vi "_script_change_copyright_year.vi"(8 "error in (no error)":errorcluster, 11 "dup path":path) -> (0 "error out":errorcluster)   [LabVIEW 2017]
uses:
  _csmHelper/CSM-Helper.lvclass/CSM-Helper.ctl
  _csmHelper/Properties/Read While Loop Ref.vi
  _csmHelper/Utility/Is CSM Module - VIRef.vi
  _csmHelper/API/Create From Basic Refs.vi
  _csmHelper/API/Open Front Panel.vi
  _csmHelper/API/Save Instrument.vi
  _csmHelper/API/Destroy.vi
  _csmHelper/Utility/CSM-Helper Utility.lvlib
  _csmHelper/CSM-Helper.lvclass
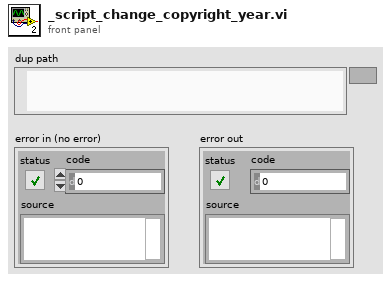
[diagram p1: front panel]
types:
  T1 = typedef "CSM-Helper Utility.lvlib/CSM Basic Refs.ctl" = cluster{"VI":refnum<vi>, "While Loop":refnum<vi>, "Case Structure":refnum<vi>, "Parse State Queue":refnum<vi>, "Event Structure":refnum<vi>, "Type":T2}
  T2 = typedef "CSM-Helper Utility.lvlib/CSM Module Type.ctl" = enum16{"Not a CSM", "JKISM", "CSM"}
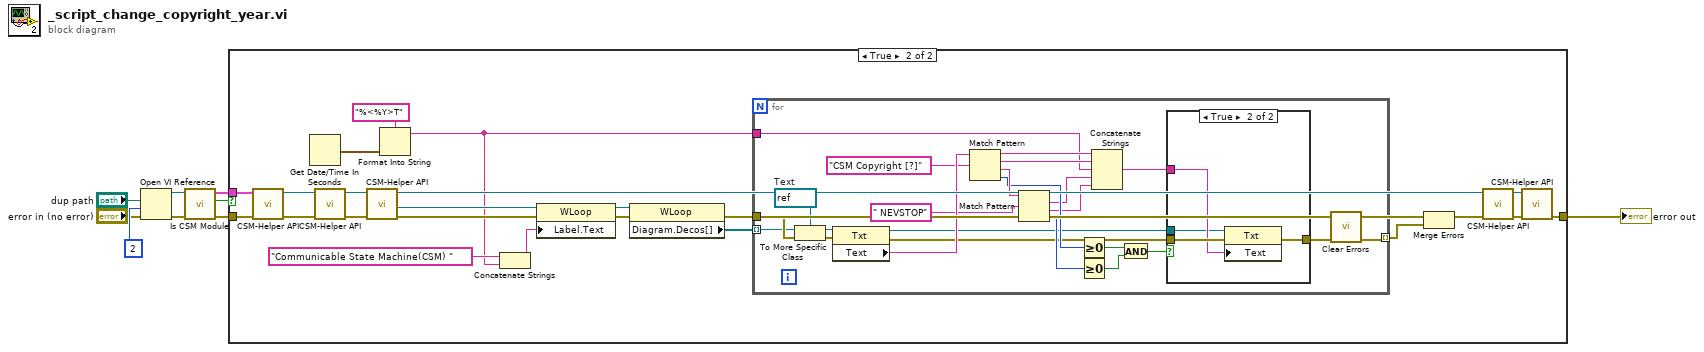
[diagram p0: block diagram]
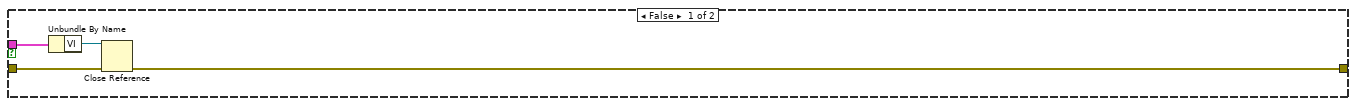
[diagram p2: hidden frame]
diagram:
  n1 = Open VI Reference(vi path="dup path", options=2, error in (no error)="error in (no error)") -> (vi reference=w6:refnum<vi>, error out=w7:errorcluster)  [unwired: 3 in]
  n2 = call-poly "Is CSM Module.vi"("error in (no error)"=w7, "VIRef"=w6) -> ("error out"=w5:errorcluster, "Is CSM Module?"=w8:bool, "CSM Basic Refs"=w4:T1)  [unwired: 7 in]
  n3 = case shown="True" w8 {
    tunnel: [w12 w36] -> w3
    tunnel: w4 -> [w11 w35]
    tunnel: w5 -> [w13 w34]
    frame False {
      n4 = Unbundle By Name(w11) -> ("VI"=w10:refnum<vi>)
      n5 = Close Reference(reference=w10, error in (no error)=w13) -> (error out=w12:errorcluster)
    }
    frame True {
      n6 = call-poly "CSM-Helper API.vi"("error in (no error)"=w34, "CSM Basic Refs"=w35) -> ("error out"=w28:errorcluster, "CSM-Helper.lvclass"=w29:refnum<class "CSM-Helper.lvclass">)  [unwired: 8 in]
      n7 = Get Date/Time In Seconds() -> (seconds since 1Jan1904=w31:timestamp)
      n8 = call-poly "CSM-Helper API.vi"("error in (no error)"=w28, "CSM-Helper in"=w29) -> ("error out"=w27:errorcluster, "CSM-Helper out"=w26:refnum<class "CSM-Helper.lvclass">)  [unwired: 8 in]
      n9 = call-poly "CSM-Helper API.vi"("error in (no error)"=w27, "CSM-Helper in"=w26) -> ("error out"=w33:errorcluster, "While Loop"=w32:refnum<vi>, "CSM-Helper out"=w22:refnum<class "CSM-Helper.lvclass">)  [unwired: 7 in]
      n10 = Format Into String(format string="%<%Y>T", w31) -> (resulting string=w14:string)  [unwired: 2 in, 1 out]
      n11 = Concatenate Strings("Communicable State Machine(CSM) " ("string"), w14) -> (w16:string)
      n12 = property class="WLoop"(reference=w32, error in=w33, "Label.Text"=w16) -> (reference out=w21:refnum<vi>, error out=w23:errorcluster)
      n13 = property class="WLoop"(reference=w21, error in=w23) -> (error out=w20:errorcluster, "Diagram.Decos[]"=w19:refnum<vi>[])  [unwired: 1 out]
      n14 = for {
        tunnel: w20 -> [w60]
        tunnel: w19 -> [w59] mode=indexing
        tunnel: [w55] -> w17 mode=indexing
        tunnel: w14 -> [w42]
        w58 = refnum<vi> refnum  # Text
        n15 = To More Specific Class(target class=w58, reference=w59, error in=w60) -> (specific class reference=w57:refnum<vi>, error out=w56:errorcluster)
        n16 = property class="Txt"(reference=w57, error in=w56) -> (reference out=w37:refnum<vi>, error out=w46:errorcluster, "Text"=w54:string)
        n17 = Match Pattern(string=w54, regular expression="CSM Copyright [?]") -> (before substring=w44:string, match substring=w43:string, after substring=w52:string, offset past match=w50:i32)  [unwired: 1 in]
        n18 = Match Pattern(string=w52, regular expression=" NEVSTOP") -> (match substring=w41:string, after substring=w40:string, offset past match=w49:i32)  [unwired: 1 in, 1 out]
        n19 = Greater Or Equal To 0?(x=w50) -> (x >= 0?=w48:bool)
        n20 = Greater Or Equal To 0?(x=w49) -> (x >= 0?=w47:bool)
        n21 = Concatenate Strings(w44, w43, w42, w41, w40) -> (w39:string)
        n22 = And(x=w48, y=w47) -> (x .and. y?=w38:bool)
        n23 = case shown="True" w38 {
          tunnel: w46 -> [w61 w65]
          tunnel: [w61 w64] -> w45
          tunnel: w39 -> [_ w63]
          tunnel: w37 -> [_ w62]
          frame False {
          }
          frame True {
            n24 = property class="Txt"(reference=w62, error in=w65, "Text"=w63) -> (error out=w64:errorcluster)  [unwired: 1 out]
          }
        }
        n25 = call <vilib>:"Clear Errors.vi"("error in (no error)"=w45) -> ("error out"=w55:errorcluster)  [unwired: 5 in, 1 out]
      }
      n26 = Merge Errors(w20, w17) -> (w18:errorcluster)
      n27 = call-poly "CSM-Helper API.vi"("error in (no error)"=w18, "CSM-Helper in"=w22) -> ("error out"=w24:errorcluster, "CSM-Helper out"=w25:refnum<class "CSM-Helper.lvclass">)  [unwired: 8 in]
      n28 = call-poly "CSM-Helper API.vi"("error in (no error)"=w24, "CSM-Helper in"=w25) -> ("error out"=w36:errorcluster)  [unwired: 8 in, 1 out]
    }
  }
  "error out" <- w3
